vi "Oxford GPIB write read.vi"(8 "error in":errorcluster, 11 "Command":string="R1") -> (0 "error out":errorcluster, 3 "Output":string)   [LabVIEW 2015]
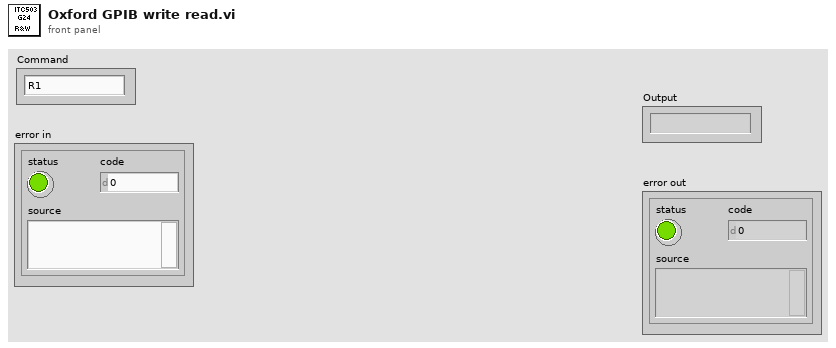
[diagram p1: front panel]
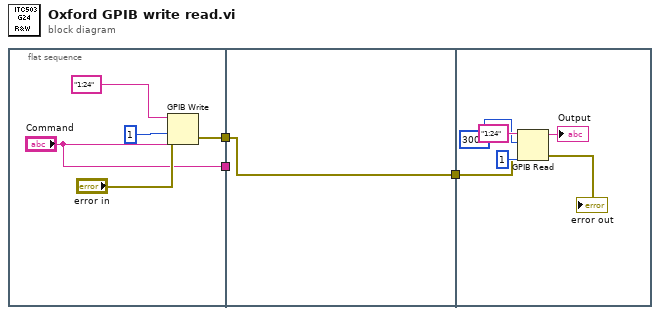
[diagram p0: block diagram]
diagram:
  n1 = flat-sequence {
    tunnel: ["Command"] -> w3
    tunnel: [w4] -> w2
    tunnel: w3 -> [_]
    tunnel: w2 -> [w9]
    tunnel: [w9] -> w1
    tunnel: w1 -> [w10]
    frame #0 {
      n2 = GPIB Write(0:"1:24" ("address string"), 1:"Command", 2:i16 1 ("mode (0)"), 3:"error in") -> (6:w4:errorcluster)  [unwired: 1 in, 1 out]
    }
    frame #1 {
    }
    frame #2 {
      n3 = GPIB Read(0:"1:24" ("address string"), 1:3000 ("byte count"), 2:i16 1 ("mode (0)"), 3:w10) -> (5:→"Output":string, 7:→"error out":errorcluster)  [unwired: 1 in, 1 out]
    }
  }
